vi "test_Scan Initilize.vi"(6 "Measure Maximun Voltage":dbl=100.0 format="%#_13g", 8 "error in (no error)":errorcluster, 9 "Current Setting":u8[](array[numeric]), 10 "Channel Count":i32, 11 "VISA Refnum in":refnum<visa-resource-name>) -> (0 "error out":errorcluster, 1 "N channel number":i32, 2 "P channel number":i32, 3 "VISA Refnum out":refnum<visa-resource-name>, 4 "Array":u32[](array[numeric]))   [LabVIEW 2023]
uses:
  <instrlib>/Agilent 3446X Series/Agilent 3446X Series.lvlib
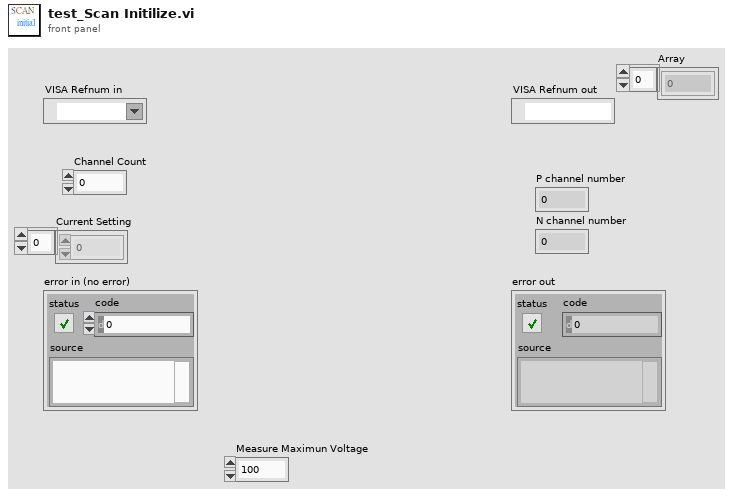
[diagram p1: front panel]
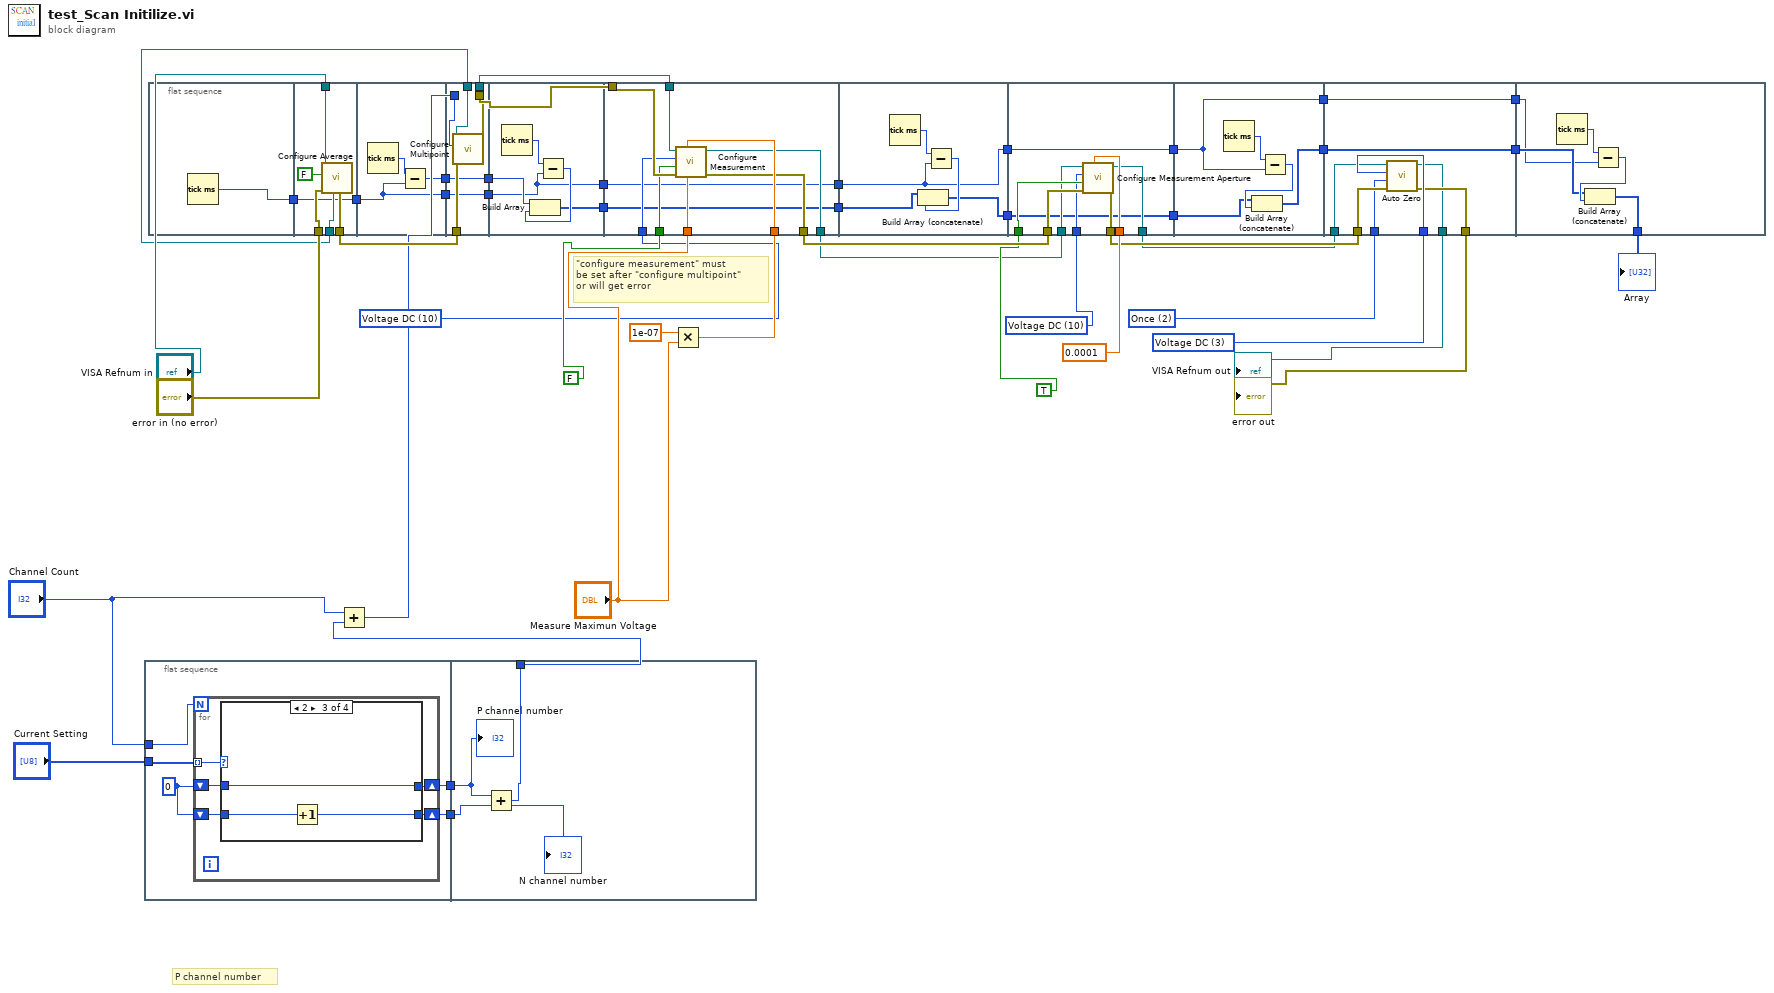
[diagram p0: block diagram]
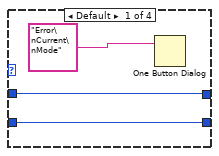
[diagram p2: hidden frame]
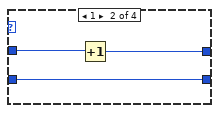
[diagram p3: hidden frame]
diagram:
  w26 = 10 items=["Continuity", "Current AC", "Current DC", "Diode", "Frequency", "Resistance 4-wire", "Period", "Resistance 2-wire", "Temperature", "Voltage AC", "Voltage DC", "Voltage DC Ratio", "Capacitance"] ("Measurement Function (10: Voltage DC)")
  w9 = 3 items=["Current DC", "Resistance", "Temperature", "Voltage DC"] ("Zero Type (0: Current DC)")
  w10 = 2 items=["Disable", "Enable", "Once"] ("Auto Zero (1: Enable)")
  w17 = 10 items=["Continuity", "Current AC", "Current DC", "Diode", "Frequency", "Resistance 4-wire", "Period", "Resistance 2-wire", "Temperature", "Voltage AC", "Voltage DC", "Voltage DC Ratio", "Capacitance"] ("Measurement Function (0: Continuity)")
  # "P channel number"
  # "\"configure measurement\" must \nbe set after \"configure multipoint\"\nor will get error"
  n1 = flat-sequence {
    tunnel: "Channel Count" -> [w52]
    tunnel: "Current Setting" -> [w51]
    tunnel: [w49] -> w46
    tunnel: [w48] -> w45
    tunnel: w46 -> [w71]
    tunnel: w45 -> [w70]
    tunnel: [w69] -> w44
    frame #0 {
      w50 = 0 ("P_current_count")
      n2 = for {
        N: w52 -> [_]
        tunnel: w51 -> [w57] mode=indexing
        shift-right: [w55] -> w49
        shift-left: w50 -> [w56]
        shift-right: [w53] -> w48
        shift-left: w50 -> [w54]
        n3 = case shown="2" w57 {
          tunnel: w56 -> [w59 w63 w64 w68]
          tunnel: [w59 w62 w64 w68] -> w55
          tunnel: w54 -> [w58 w61 w66 w67]
          tunnel: [w58 w61 w65 w67] -> w53
          frame Default {
            n4 = One Button Dialog(message="Error\nCurrent\nMode" ("error source (\" \")")) -> ()  [unwired: 1 in, 1 out]
          }
          frame 1 {
            n5 = Increment(x=w63) -> (x+1=w62:i32)
          }
          frame 2 {
            n6 = Increment(x=w66) -> (x+1=w65:i32)
          }
          frame 0 {
          }
        }
      }
    }
    frame #1 {
      n7 = Add(x=w71, y=w70) -> (x+y=w69:i32)
      "P channel number" <- w71
      "N channel number" <- w70
    }
  }
  n8 = flat-sequence {
    tunnel: [w72] -> w39
    tunnel: "error in (no error)" -> [w78]
    tunnel: "VISA Refnum in" -> [w76]
    tunnel: [w75] -> w37
    tunnel: [w74] -> w35
    tunnel: w39 -> [w73]
    tunnel: [w73] -> w38
    tunnel: w38 -> [w80]
    tunnel: [w80] -> w34
    tunnel: [w79] -> w32
    tunnel: w37 -> [w88]
    tunnel: w36 -> [w87]
    tunnel: w35 -> [w86]
    tunnel: [w85] -> w28
    tunnel: [w84] -> w25
    tunnel: w34 -> [w83]
    tunnel: [w83] -> w33
    tunnel: w32 -> [w82]
    tunnel: [w82] -> w31
    tunnel: w33 -> [w89]
    tunnel: w31 -> [w92]
    tunnel: [w90] -> w24
    tunnel: [w89] -> w22
    tunnel: "Measure Maximun Voltage" -> [w103]
    tunnel: w29 -> [w102]
    tunnel: w28 -> [w101]
    tunnel: FALSE ("Auto Range (T: Enable)") -> [w100]
    tunnel: w26 -> [w99]
    tunnel: w25 -> [w98]
    tunnel: [w97] -> w19
    tunnel: [w96] -> w16
    tunnel: w24 -> [w95]
    tunnel: [w95] -> w23
    tunnel: w22 -> [w94]
    tunnel: [w94] -> w21
    tunnel: w23 -> [w105]
    tunnel: w21 -> [w106]
    tunnel: [w106] -> w15
    tunnel: [w104] -> w13
    tunnel: 0.0001 ("Aperture Time (0.1s)") -> [w117]
    tunnel: w19 -> [w116]
    tunnel: TRUE ("Enable Aperture (F: Disable)") -> [w115]
    tunnel: w17 -> [w114]
    tunnel: w16 -> [w113]
    tunnel: [w112] -> w11
    tunnel: [w111] -> w8
    tunnel: w15 -> [w110]
    tunnel: [w110] -> w14
    tunnel: w13 -> [w109]
    tunnel: [w109] -> w12
    tunnel: w14 -> [w118]
    tunnel: w12 -> [w120]
    tunnel: [w119] -> w4
    tunnel: [w118] -> w3
    tunnel: w11 -> [w130]
    tunnel: w10 -> [w129]
    tunnel: w9 -> [w128]
    tunnel: w8 -> [w127]
    tunnel: [w126] -> w7
    tunnel: [w125] -> w6
    tunnel: [w124] -> w5
    tunnel: w4 -> [w124]
    tunnel: w3 -> [w123]
    tunnel: [w123] -> w2
    tunnel: w5 -> [w133]
    tunnel: w2 -> [w132]
    tunnel: [w131] -> w1
    frame #0 {
      n9 = Tick Count (ms)() -> (millisecond timer value=w72:u32)
    }
    frame #1 {
      n10 = call <instrlib>:"Configure Average.vi"("error in (no error)"=w78, "Enable Statistics (F: Disable)"=FALSE, "VISA resource name"=w76) -> ("error out"=w75:errorcluster, "VISA resource name out"=w74:refnum<visa-resource-name>)  [unwired: 7 in]
    }
    frame #2 {
      n11 = Tick Count (ms)() -> (millisecond timer value=w81:u32)
      n12 = Subtract(x=w81, y=w80) -> (x-y=w79:u32)
    }
    frame #3 {
      n13 = call <instrlib>:"Configure Multipoint.vi"("error in (no error)"=w88, "Trigger Count (1)"=w87, "VISA resource name"=w86) -> ("error out"=w85:errorcluster, "VISA resource name out"=w84:refnum<visa-resource-name>)  [unwired: 4 in, 3 out]
    }
    frame #4 {
      n14 = Tick Count (ms)() -> (millisecond timer value=w93:u32)
      n15 = Subtract(x=w93, y=w89) -> (x-y=w91:u32)
      n16 = Build Array(w92, w91) -> (w90:u32[])
    }
    frame #5 {
      n17 = call <instrlib>:"Configure Measurement.vi"("Manual Range (1)"=w103, "Absolute Resolution (1E-6)"=w102, "error in (no error)"=w101, "Auto Range (T: Enable)"=w100, "Measurement Function (10: Voltage DC)"=w99, "VISA resource name"=w98) -> ("error out"=w97:errorcluster, "VISA resource name out"=w96:refnum<visa-resource-name>)  [unwired: 4 out]
    }
    frame #6 {
      n18 = Tick Count (ms)() -> (millisecond timer value=w108:u32)
      n19 = Subtract(x=w108, y=w106) -> (x-y=w107:u32)
      n20 = Build Array (concatenate)(w105, w107) -> (w104:u32[])
    }
    frame #7 {
      n21 = call <instrlib>:"Configure Measurement Aperture.vi"("Aperture Time (0.1s)"=w117, "error in (no error)"=w116, "Enable Aperture (F: Disable)"=w115, "Measurement Function (0: Continuity)"=w114, "VISA resource name"=w113) -> ("error out"=w112:errorcluster, "VISA resource name out"=w111:refnum<visa-resource-name>)  [unwired: 5 in]
    }
    frame #8 {
      n22 = Tick Count (ms)() -> (millisecond timer value=w122:u32)
      n23 = Subtract(x=w122, y=w118) -> (x-y=w121:u32)
      n24 = Build Array (concatenate)(w120, w121) -> (w119:u32[])
    }
    frame #9 {
      n25 = call <instrlib>:"Auto Zero.vi"("error in (no error)"=w130, "Auto Zero (1: Enable)"=w129, "Zero Type (0: Current DC)"=w128, "VISA resource name"=w127) -> ("error out"=w126:errorcluster, "VISA resource name out"=w125:refnum<visa-resource-name>)  [unwired: 6 in]
    }
    frame #10 {
      n26 = Tick Count (ms)() -> (millisecond timer value=w135:u32)
      n27 = Subtract(x=w135, y=w132) -> (x-y=w134:u32)
      n28 = Build Array (concatenate)(w133, w134) -> (w131:u32[])
    }
  }
  n29 = Add(x="Channel Count", y=w44) -> (x+y=w36:i32)
  n30 = Multiply(x=1e-07, y="Measure Maximun Voltage") -> (x*y=w29:dbl)
  "error out" <- w7
  "VISA Refnum out" <- w6
  "Array" <- w1
